vi "Get States.vi"(8 "error in (no error)":errorcluster, 11 "Example App Properties in":refnum<class "Example App Properties.lvclass">) -> (0 "error out":errorcluster, 2 "UUT States":T1[](array[typedef]), 3 "Example App Properties out":refnum<class "Example App Properties.lvclass">)   [LabVIEW 2015, in "Example Application.lvlib" / "Example App Properties.lvclass"]
uses:
  Example App Properties.lvclass
  DUT State -- Enum.ctl
  Example App Properties.lvclass/Example App Properties.ctl
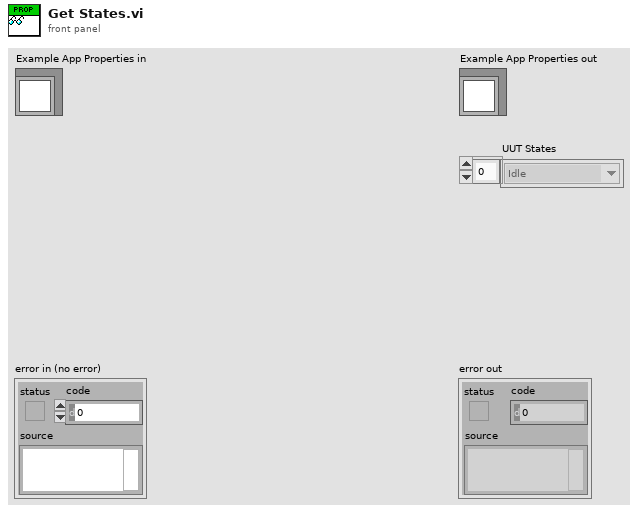
[diagram p1: front panel]
types:
  T1 = typedef "Example Application.lvlib/Example App Properties.lvclass/DUT State -- Enum.ctl" = enum16{"Idle", "Testing", "Passed", "Failed"}
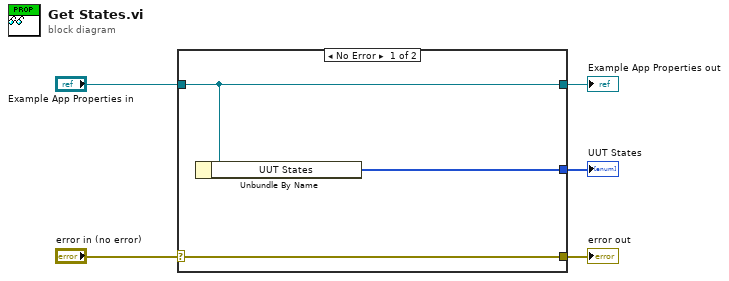
[diagram p0: block diagram]
diagram:
  n1 = case shown="No Error" "error in (no error)" {
    selector: "error in (no error)" -> [w8 w9]
    tunnel: [w8 w9] -> w4
    tunnel: [w7 w10] -> w2
    tunnel: "Example App Properties in" -> [w7 w10]
    tunnel: [w6 _] -> w1
    frame No Error {
      n2 = Unbundle By Name(w7) -> ("UUT States"=w6:T1[])
    }
    frame Error {
    }
  }
  "error out" <- w4
  "Example App Properties out" <- w2
  "UUT States" <- w1
